vi "controlContinousFwd.vi"(7 "Set":bool, 8 "error in":errorcluster, 9 "continous FWD in":bool=TRUE, 10 "axis in":u8, 11 "connection ID":i32) -> (0 "error out":errorcluster, 1 "continous FWD out":bool=TRUE, 2 "axis out":u8, 3 "connection ID":i32)   [LabVIEW 2016]
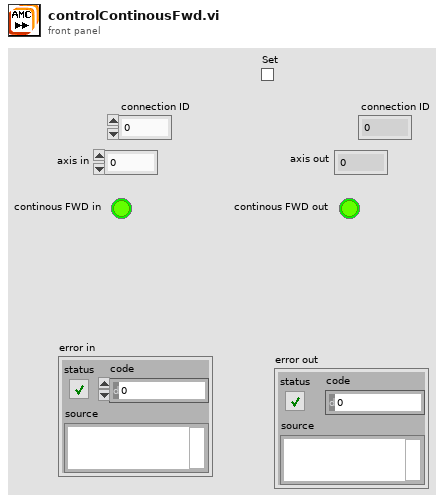
[diagram p1: front panel]
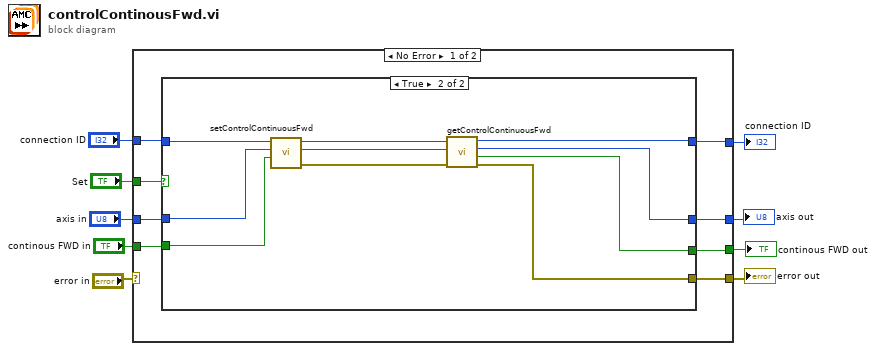
[diagram p0: block diagram]
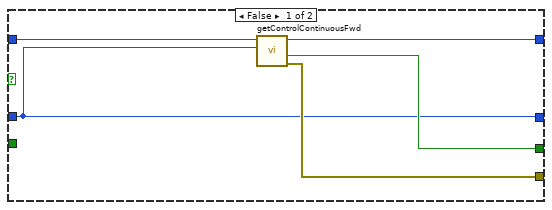
[diagram p2: hidden frame]
diagram:
  n1 = case shown="No Error" "error in" {
    selector: "error in" -> [_ w36]
    tunnel: "axis in" -> [w14 w34]
    tunnel: [w10 w36] -> w8
    tunnel: [w12 w34] -> w7
    tunnel: "Set" -> [w16 _]
    tunnel: [w11 w35] -> w5
    tunnel: "continous FWD in" -> [w15 w35]
    tunnel: [w13 w33] -> w3
    tunnel: "connection ID" -> [w17 w33]
    frame No Error {
      n2 = case shown="True" w16 {
        tunnel: [w21 w28] -> w13
        tunnel: w17 -> [w22 w32]
        tunnel: w14 -> [w18 w30]
        tunnel: [w18 w27] -> w12
        tunnel: [w19 w26] -> w11
        tunnel: [w20 w25] -> w10
        tunnel: w15 -> [_ w31]
        frame False {
          n3 = call "getControlContinuousFwd.vi"("axis"=w18, "connection ID"=w22) -> ("error out"=w20:errorcluster, "enabled"=w19:bool, "connection ID"=w21:i32)  [unwired: 6 in, 1 out]
        }
        frame True {
          n4 = call "setControlContinuousFwd.vi"("enable"=w31, "axis"=w30, "connection ID"=w32) -> ("error out"=w24:errorcluster, "axis_out"=w23:i32, "connection ID"=w29:i32)  [unwired: 6 in]
          n5 = call "getControlContinuousFwd.vi"("error in"=w24, "axis"=w23, "connection ID"=w29) -> ("error out"=w25:errorcluster, "enabled"=w26:bool, "axis_out"=w27:i32, "connection ID"=w28:i32)  [unwired: 5 in]
        }
      }
    }
    frame Error {
    }
  }
  "error out" <- w8
  "axis out" <- w7
  "continous FWD out" <- w5
  "connection ID" <- w3
